vi "Serial.vi"() -> ()   [LabVIEW 2022 SP3]
doc: "The Simple Serial VI performs a Serial Port Read, a Serial Port Write, or closes the serial port, or a combination of these actions. The user selects the actions (read, write or close) on the front panel."
uses:
  <vilib>/Instr/_visa.llb/VISA Configure Serial Port (Instr).vi
panel:
  in  "Stop":bool
  in  "Write (T)":bool
  in  "Close":bool
  in  "Resource Name":refnum<visa-resource-name>="ASRL1::INSTR"
  out "Error Information":errorcluster
  out "Bytes to Read":u32=5
  out "Read String":string
  in  "String To Write":string="Sample String to read"
  # "If the VISA Session is not closed \nwhen communications are finished,  \nnon VISA communications with the \nport may not be possible."
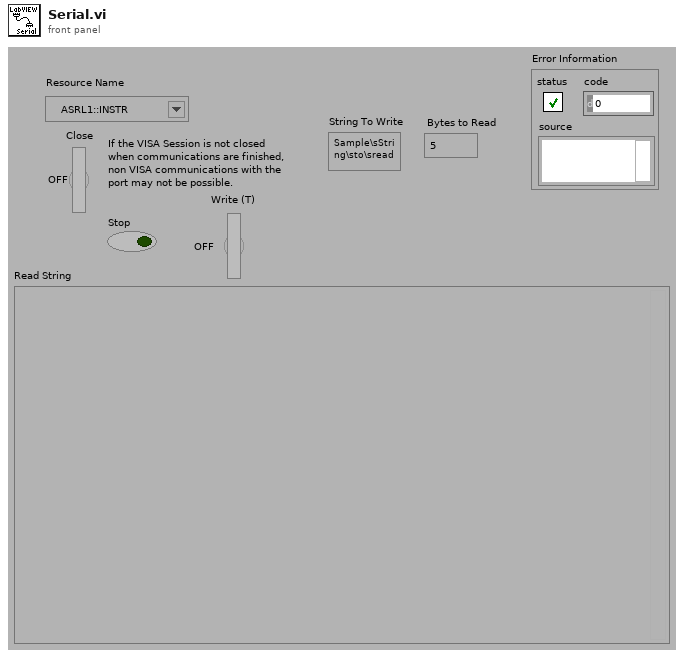
[diagram p1: front panel]
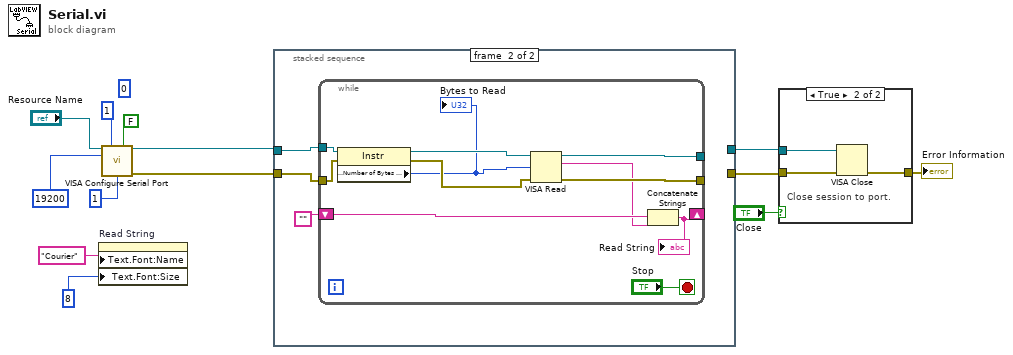
[diagram p0: block diagram]
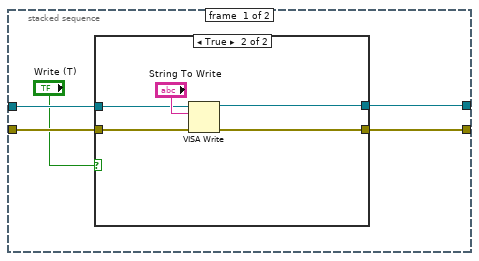
[diagram p2: hidden frame]
diagram:
  (unwired) 0
  n1 = property on="Read String" class="Str"("Text.Font:Name"="Courier", "Text.Font:Size"=8) -> ()  [unwired: 2 in, 2 out]
  n2 = call-poly "VISA Configure Serial Port"("VISA resource name"="Resource Name", "timeout (10sec)"=1, "Enable Termination\nChar (T)"=FALSE, "baud rate (9600)"=u32 19200 ("Baud Rate (9600)"), "flow control (0:none)"=1) -> ("VISA resource name out"=w6:refnum<visa-resource-name>, "error out"=w5:errorcluster)  [unwired: 3 in, 6 out]
  n3 = stacked-sequence {
    tunnel: w5 -> [w17 w28]
    tunnel: w6 -> [w18 w27]
    tunnel: [w15 _] -> w11
    tunnel: [w16 _] -> w9
    frame #0 {
      n4 = case shown="True" "Write (T)" {
        tunnel: w18 -> [w20 w24]
        tunnel: w17 -> [w19 w23]
        tunnel: [w20 w22] -> w16
        tunnel: [w19 w21] -> w15
        frame False {
        }
        frame True {
          n5 = VISA Write(VISA resource name=w24, write buffer="String To Write", error in (no error)=w23) -> (VISA resource name out=w22:refnum<visa-resource-name>, error out=w21:errorcluster)  [unwired: 1 out]
        }
      }
    }
    frame #1 {
      n6 = while {
        tunnel: w28 -> [w29]
        tunnel: w27 -> [w38]
        tunnel: [w36] -> _
        tunnel: [w35] -> _
        shift-right: [w31] -> _
        shift-left: "" -> [w33]
        stop <- "Stop" stop-if-true
        n7 = property class="Instr"(reference=w38, error in=w29) -> (reference out=w39:refnum<visa-resource-name>, error out=w37:errorcluster, "Serial Settings:Number of Bytes at Serial Port"=w34:u32)
        "Bytes to Read" <- w34
        n8 = VISA Read(VISA resource name=w39, byte count=w34, error in (no error)=w37) -> (VISA resource name out=w35:refnum<visa-resource-name>, read buffer=w32:string, error out=w36:errorcluster)  [unwired: 1 out]
        n9 = Concatenate Strings(w33, w32) -> (w31:string)
        "Read String" <- w31
      }
    }
  }
  n10 = case shown="True" "Close" {
    tunnel: w9 -> [_ w43]
    tunnel: w11 -> [w40 w42]
    tunnel: [w40 w41] -> w10
    frame False {
    }
    frame True {
      # "Close session to port."
      n11 = VISA Close(VISA resource name=w43, error in (no error)=w42) -> (error out=w41:errorcluster)
    }
  }
  "Error Information" <- w10
